vi "VISA.vi"(8 "error in (no error)":errorcluster, 11 "AOTF in":refnum<class "Invivo_AOTF.lvclass">) -> (0 "error out":errorcluster, 3 "AOTF out":refnum<class "Invivo_AOTF.lvclass">)   [LabVIEW 2012, in "Invivo_AOTF.lvclass"]
uses:
  Invivo_AOTF.lvclass
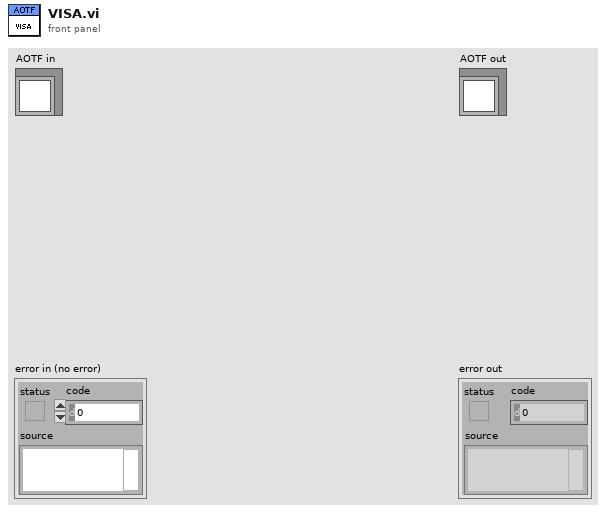
[diagram p1: front panel]
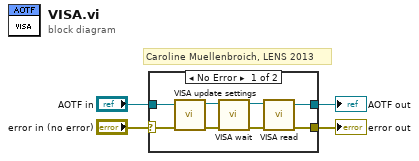
[diagram p0: block diagram]
diagram:
  # "Caroline Muellenbroich, LENS 2013"
  n1 = case shown="No Error" "error in (no error)" {
    selector: "error in (no error)" -> [w8 w14]
    tunnel: [w7 w14] -> w3
    tunnel: [w5 w13] -> w1
    tunnel: "AOTF in" -> [w6 w13]
    frame No Error {
      n2 = call-dynamic "VISA update settings.vi"("error in (no error)"=w8, "AOTF in"=w6) -> ("error out"=w10:errorcluster, "AOTF out"=w9:refnum<class "Invivo_AOTF.lvclass">)  [unwired: 8 in]
      n3 = call-dynamic "VISA wait.vi"("error in (no error)"=w10, "AOTF in"=w9) -> ("error out"=w12:errorcluster, "AOTF out"=w11:refnum<class "Invivo_AOTF.lvclass">)  [unwired: 8 in]
      n4 = call-dynamic "VISA read.vi"("error in (no error)"=w12, "AOTF in"=w11) -> ("error out"=w7:errorcluster, "AOTF out"=w5:refnum<class "Invivo_AOTF.lvclass">)  [unwired: 7 in, 1 out]
    }
    frame Error {
    }
  }
  "error out" <- w3
  "AOTF out" <- w1
